vi "UDP Set Last Update Channel.vi"(8 "error in (no error)":errorcluster, 10 "TBM channel in":refnum<class "TBM channel.lvclass">, 11 "Node Ref":refnum<data-value>) -> (0 "error out":errorcluster, 3 "E2E editor node out":refnum<data-value>)   [LabVIEW 2015, in "E2E Tag Exchange editor node.lvclass"]
uses:
  E2E Tag Exchange editor node.lvclass
  <vilib>/NI/Tag Bus Module Framework/channel/TBM channel.lvclass
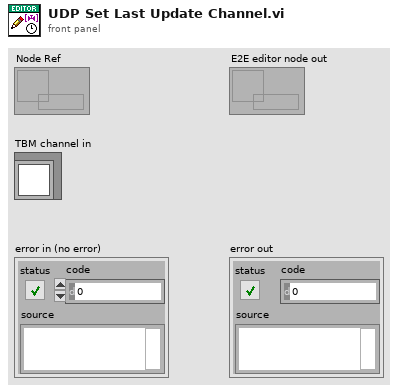
[diagram p1: front panel]
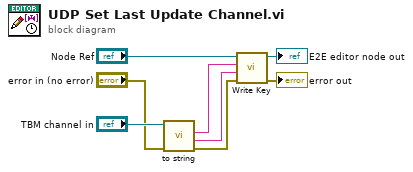
[diagram p0: block diagram]
diagram:
  n1 = call-dynamic "to string.vi"("error in"="error in (no error)", "channel in"="TBM channel in") -> ("error out"=w1:errorcluster, "channel data"=w7:string, "identifier"=w6:string)  [unwired: 6 in, 1 out]
  n2 = call "Write Key.vi"("error in (no error)"=w1, "Value"=w7, "Key"=w6, "E2E editor node in"="Node Ref") -> ("error out"=→"error out":errorcluster, "E2E editor node out"=→"E2E editor node out":refnum<data-value>)  [unwired: 6 in]
